vi "LVClass_WavefrontCorrector Check Relative Position.vi"(0 "WavefrontCorrector in":refnum<class "WavefrontCorrector.lvclass">, 5 "Relative Positions":T1, 11 "error in (no error)":errorcluster) -> (4 "WavefrontCorrector out":refnum<class "WavefrontCorrector.lvclass">, 6 "Relative Positions OUT":T1, 15 "error out":errorcluster)   [LabVIEW 2020, in "WavefrontCorrector.lvclass"]
doc: "Assert if requested relative positions satisfy current preferences.\n\n--------------------------------------------------------------------------------\n\n<B>correctorIn </B> : WavefrontCorrector object.\n<B>correctorOut </B> : WavefrontCorrector object.\n<B>position </B> : Requested relatives positions.\n<B>ErrorIn </B> : Error\n<B>ErrorOut </B> : Error\n\n--------------------------------------------------------------------------------"
uses:
  WavefrontCorrector.lvclass
  Wavefront Corrector Position.ctl
  WavefrontCorrector.lvclass/WavefrontCorrector.ctl
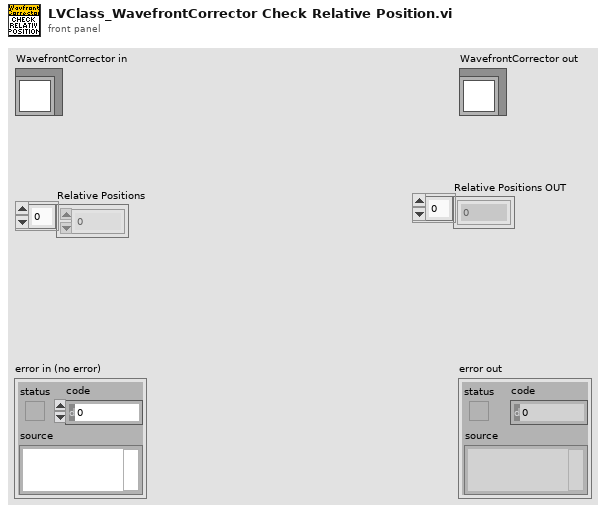
[diagram p1: front panel]
types:
  T1 = typedef "Wavefront Corrector Position.ctl" = sgl[]
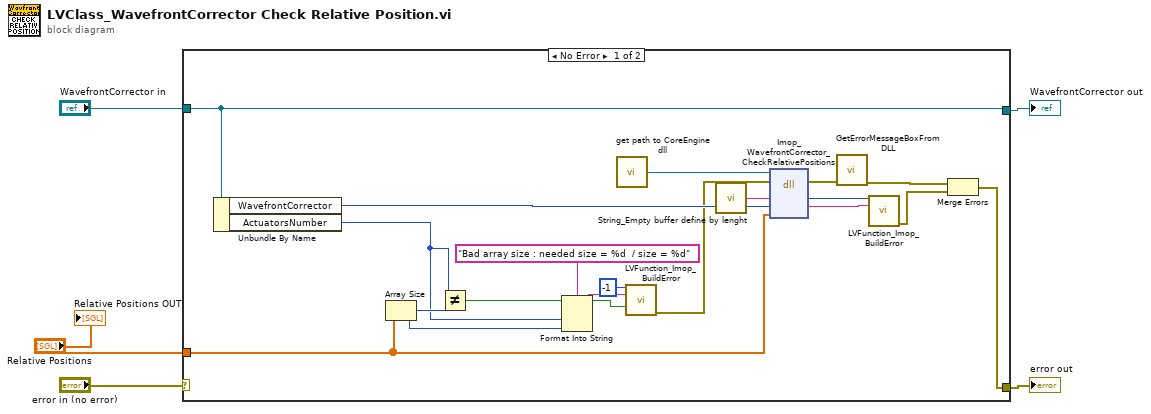
[diagram p0: block diagram]
diagram:
  n1 = case shown="No Error" "error in (no error)" {
    selector: "error in (no error)" -> [_ w25]
    tunnel: [w15 w25] -> w2
    tunnel: [w14 w24] -> w3
    tunnel: "WavefrontCorrector in" -> [w14 w24]
    tunnel: "Relative Positions" -> [w6 _]
    frame No Error {
      n2 = Unbundle By Name(w14) -> ("WavefrontCorrector"=w16:i32, "ActuatorsNumber"=w8:i32)
      n3 = Array Size(array=w6) -> (size(s)=w11:i32)
      n4 = Not Equal?(x=w8, y=w11) -> (x != y?=w10:bool)
      n5 = Format Into String(format string="Bad array size : needed size = %d  / size = %d" ("String to Prepend to source (\"\")"), w8, w11) -> (resulting string=w12:string)  [unwired: 2 in, 1 out]
      n6 = call "get path to CoreEngine dll.vi"() -> ("path to c_interface_vc100.dll"=w20:path)  [unwired: 12 in, 3 out]
      n7 = call "LVFunction_Imop_BuildError.vi"("code"=-1, "String to Prepend to source (\"\")"=w12, "Activate error? (true)"=w10) -> ("error out"=w7:errorcluster)  [unwired: 12 in]
      n8 = call "String_Empty buffer define by lenght.vi"() -> ("Empty buffer"=w21:string)  [unwired: 1 in]
      n9 = dll-call lib="D:/soft/HASO_v3/SVN_trunk/ImOpCoreEngine4_LV2011/DLLs/c_interface_vc100.dll" fn="Imop_WavefrontCorrector_CheckRelativePositions"(path in=w20, error in=w7, "message"=w21, "WavefrontCorrection"=w16, "Relative Position"=w6) -> (error out=w19:errorcluster, "return type"=w23:i32, "message"=w22:string)  [unwired: 3 in, 1 out]
      n10 = call "GetErrorMessageBoxFromDLL.vi"("error IN"=w19) -> ("error OUT"=w18:errorcluster)  [unwired: 10 in]
      n11 = call "LVFunction_Imop_BuildError.vi"("code"=w23, "String to Prepend to source (\"\")"=w22) -> ("error out"=w17:errorcluster)  [unwired: 13 in]
      n12 = Merge Errors(w18, w17) -> (w15:errorcluster)
    }
    frame Error {
    }
  }
  "error out" <- w2
  "WavefrontCorrector out" <- w3
  "Relative Positions OUT" <- "Relative Positions"
